vi "new_series.vi"(8 "error in (no error)":errorcluster, 10 "output cluster":T1, 11 "series_class in":refnum<class "series_class.lvclass">) -> (0 "error out":errorcluster, 3 "series_class out":refnum<class "series_class.lvclass">)   [LabVIEW 2024, in "series_class.lvclass"]
uses:
  series_class.lvclass
  definitions/seriesJSON.ctl
  definitions/seriesInfo.ctl
  definitions/issueInfo.ctl
  definitions/creator.ctl
  definitions/character.ctl
  definitions/team.ctl
  definitions/location.ctl
  definitions/concept.ctl
  definitions/thing.ctl
  definitions/storyArc.ctl
  series_class.lvclass/series_class.ctl
  issue_class/issue_class.lvclass
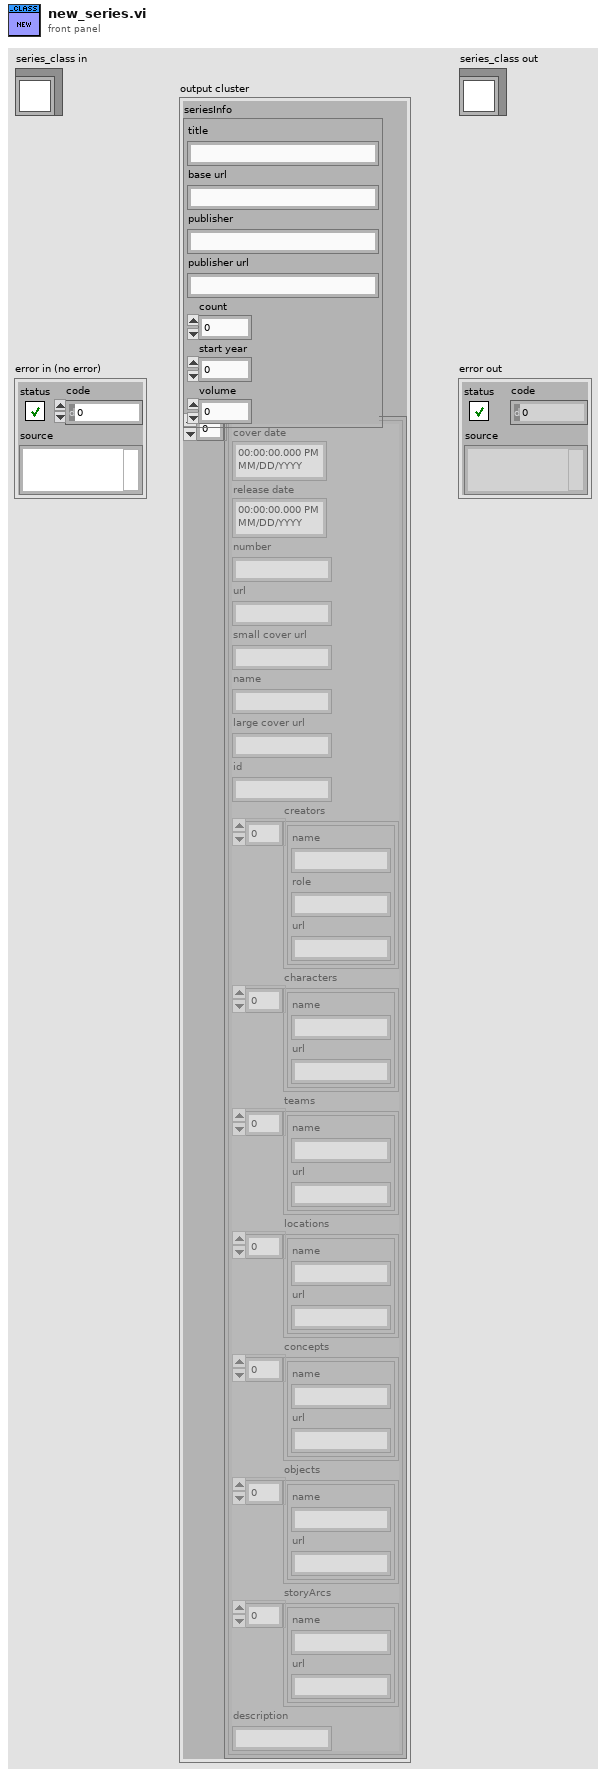
[diagram p1: front panel]
types:
  T1 = typedef "seriesJSON.ctl" = cluster{"seriesInfo":T2, "issueInfo":T3[]}
  T2 = typedef "seriesInfo.ctl" = cluster{"title":string, "base url":string, "publisher":string, "publisher url":string, "count":i32, "start year":i32, "volume":i32}
  T3 = typedef "issueInfo.ctl" = cluster{"cover date":timestamp, "release date":timestamp, "number":string, "url":string, "small cover url":string, "name":string, "large cover url":string, "id":string, "creators":T4[], "characters":T5[], "teams":T6[], "locations":T7[], "concepts":T8[], "objects":T9[], "storyArcs":T10[], "description":string}
  T4 = typedef "creator.ctl" = cluster{"name":string, "role":string, "url":string}
  T5 = typedef "character.ctl" = cluster{"name":string, "url":string}
  T6 = typedef "team.ctl" = cluster{"name":string, "url":string}
  T7 = typedef "location.ctl" = cluster{"name":string, "url":string}
  T8 = typedef "concept.ctl" = cluster{"name":string, "url":string}
  T9 = typedef "thing.ctl" = cluster{"name":string, "url":string}
  T10 = typedef "storyArc.ctl" = cluster{"name":string, "url":string}
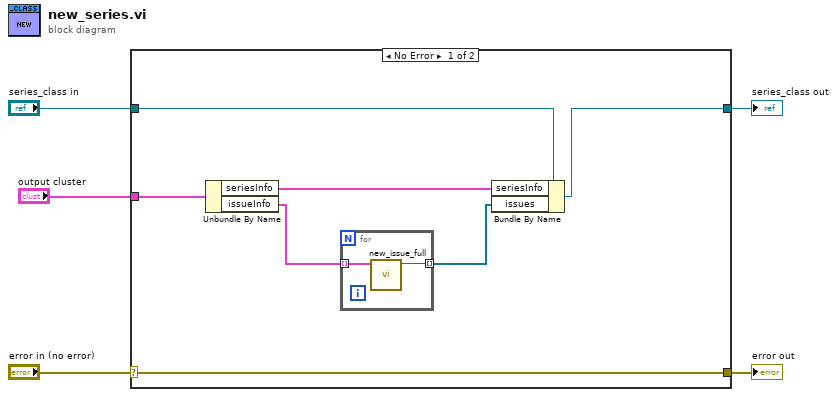
[diagram p0: block diagram]
diagram:
  n1 = case shown="No Error" "error in (no error)" {
    selector: "error in (no error)" -> [w12 w16]
    tunnel: [w12 w16] -> w4
    tunnel: [w10 w15] -> w2
    tunnel: "series_class in" -> [w11 w15]
    tunnel: "output cluster" -> [w9 _]
    frame No Error {
      n2 = Unbundle By Name(w9) -> ("seriesInfo"=w8:T2, "issueInfo"=w7:T3[])
      n3 = for {
        tunnel: w7 -> [w14] mode=indexing
        tunnel: [w13] -> w6 mode=indexing
        n4 = call "new_issue_full.vi"("issueInfo"=w14) -> ("issue_class out"=w13:refnum<class "issue_class.lvclass">)  [unwired: 10 in]
      }
      n5 = Bundle By Name(cluster=w11, "seriesInfo"=w8, "issues"=w6) -> (w10:refnum<class "series_class.lvclass">)
    }
    frame Error {
    }
  }
  "error out" <- w4
  "series_class out" <- w2
